vi "check_relay.vi"(1 "Wait (ms)":i32=100, 2 "Relay Status":bool, 3 "Relay":i32=1 min=1 max=12, 4 "Slot":i32=10 min=0 max=14) -> (0 "success":bool)   [LabVIEW 2011]
panel:
  out "elapsed":i32
  out "done":bool
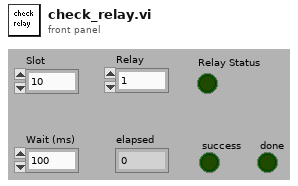
[diagram p1: front panel]
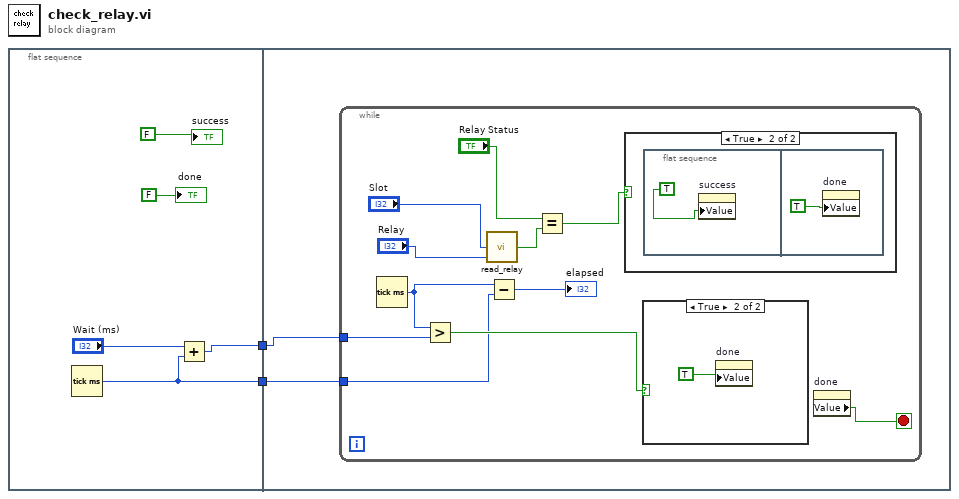
[diagram p0: block diagram]
diagram:
  n1 = flat-sequence {
    tunnel: [w7] -> w2
    tunnel: [w4] -> w1
    tunnel: w2 -> [w9]
    tunnel: w1 -> [w8]
    frame #0 {
      n2 = Tick Count (ms)() -> (millisecond timer value=w4:u32)
      n3 = Add(x="Wait (ms)", y=w4) -> (x+y=w7:u32)
      "success" <- FALSE
      "done" <- FALSE ("done")
    }
    frame #1 {
      n4 = while {
        tunnel: w9 -> [w19]
        tunnel: w8 -> [w11]
        stop <- w15 stop-if-true
        n5 = Tick Count (ms)() -> (millisecond timer value=w12:u32)
        n6 = Greater?(x=w12, y=w19) -> (0:w13:bool)
        n7 = call "read_relay.vi"("Relay"="Relay", "Slot"="Slot") -> ("Relay Status"=w20:bool)  [unwired: 1 out]
        n8 = Subtract(x=w12, y=w11) -> (x-y=→"elapsed":u32)
        n9 = Equal?(x="Relay Status", y=w20) -> (x = y?=w14:bool)
        n10 = case shown="True" w14 {
          frame False {
          }
          frame True {
            n11 = flat-sequence {
              frame #0 {
                n12 = property on="success" class="Bool (strict)"("Value"=TRUE ("success 2")) -> ()  [unwired: 2 in, 2 out]
              }
              frame #1 {
                n13 = property on="done" class="Bool (strict)"("Value"=TRUE ("done")) -> ()  [unwired: 2 in, 2 out]
              }
            }
          }
        }
        n14 = case shown="True" w13 {
          frame False {
          }
          frame True {
            n15 = property on="done" class="Bool (strict)"("Value"=TRUE) -> ()  [unwired: 2 in, 2 out]
          }
        }
        n16 = property on="done" class="Bool (strict)"() -> ("Value"=w15:bool)  [unwired: 2 in, 2 out]
      }
    }
  }
